vi "读TDM文件.vi"() -> ()   [LabVIEW 2010]
doc: "Reads a TDM (Test Data Exchange Format) file."
uses:
  <vilib>/Platform/storage/lvStorage.llb/xStorage/Open Data Storage/Open Data Storage.xnode
  <vilib>/Platform/storage/lvStorage.llb/_openFunction.ctl
  <vilib>/Platform/storage/lvStorage.llb/xStorage/Read Data/Read Data.xnode
  <vilib>/Platform/storage/lvStorage.llb/xStorage/Close Data Storage/Close Data Storage.xnode
  <vilib>/Platform/storage/lvStorage.llb/_openStorageWithRootAutoDetect.vi
  <vilib>/Platform/storage/lvStorage.llb/_queryPropString.vi
  <vilib>/Platform/storage/lvStorage.llb/_queryGenericObjects.vi
  <vilib>/Platform/storage/lvStorage.llb/_loadAllDouble.vi
  <vilib>/Platform/storage/Storage.llb/Get Object Info.vi
  <vilib>/Platform/storage/Storage.llb/__closeStorageFromObject.vi
panel:
  out "波形图":dbl[][](graph)
  in  "路径":path=path "F:/c7/prog7/lvt.tdm"
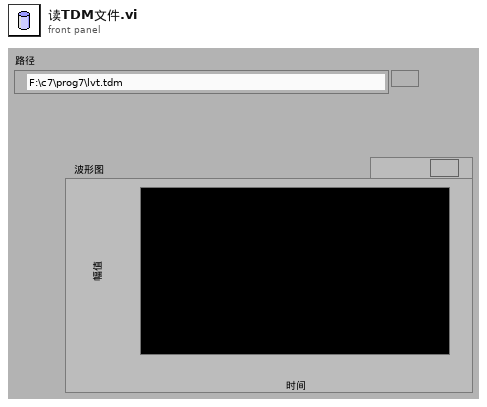
[diagram p1: front panel]
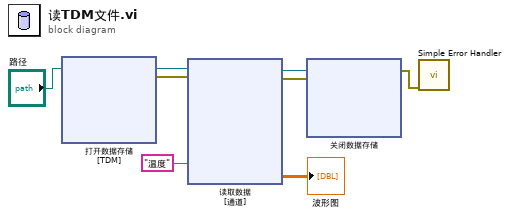
[diagram p0: block diagram]
diagram:
  n1 = xnode "打开数据存储\n[TDM]"("文件路径"="路径") -> ("存储引用句柄（文件）"=w5:refnum<k20>, "错误输出"=w7:errorcluster)  [unwired: 4 in, 1 out]
  n2 = xnode "读取数据\n[通道]"("名称"="温度", "存储引用句柄（文件）"=w5, "错误输入"=w7) -> ("信号"=→"波形图":dbl[][], "存储引用句柄（文件） 输出"=w3:refnum<k20>, "错误输出"=w2:errorcluster)  [unwired: 1 out]
  n3 = xnode "关闭数据存储\n"("存储引用句柄（文件）"=w3, "错误输入（无错误）"=w2) -> ("错误输出"=w8:errorcluster)  [unwired: 1 out]
  n4 = call <vilib>:"Simple Error Handler.vi"("error in (no error)"=w8) -> ()  [unwired: 4 in, 5 out]
